vi "Get Waveform Subset.vi"(8 "error in (no error)":errorcluster, 9 "Index B":u16, 10 "Index A":u16, 11 "Waveform":dbl[](array[numeric])) -> (0 "error out":errorcluster, 3 "Waveform Subset":dbl[](array[numeric]))   [LabVIEW 2015, in "Fuel Injection Addon Engine.lvlib"]
uses:
  Fuel Injection Addon Engine.lvlib
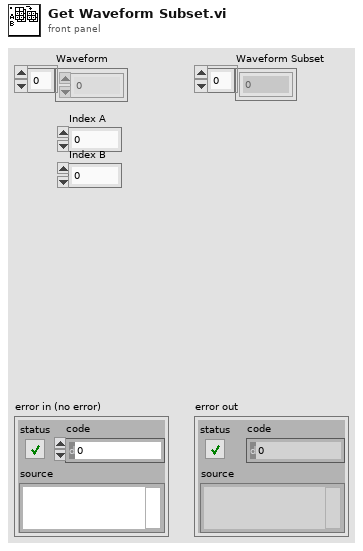
[diagram p1: front panel]
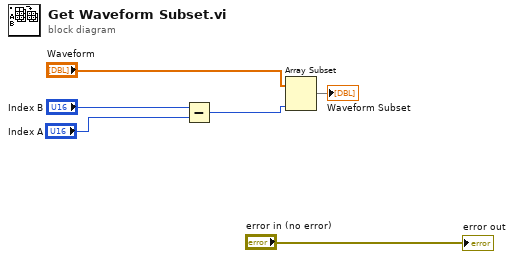
[diagram p0: block diagram]
diagram:
  n1 = Subtract(x="Index B", y="Index A") -> (x-y=w4:u16)
  n2 = Array Subset(array="Waveform", length=w4) -> (→"Waveform Subset":dbl[])  [unwired: 1 in]
  "error out" <- "error in (no error)"
